vi "Operate.vi"(8 "error in (no error)":errorcluster, 11 "Multiply in":refnum<class "Multiply.lvclass">) -> (0 "error out":errorcluster, 2 "C":dbl, 3 "Multiply out":refnum<class "Multiply.lvclass">)   [LabVIEW 2021, in "Calculator.lvlib" / "Multiply.lvclass"]
doc: "This VI is a method for multiply class."
uses:
  Multiply.lvclass
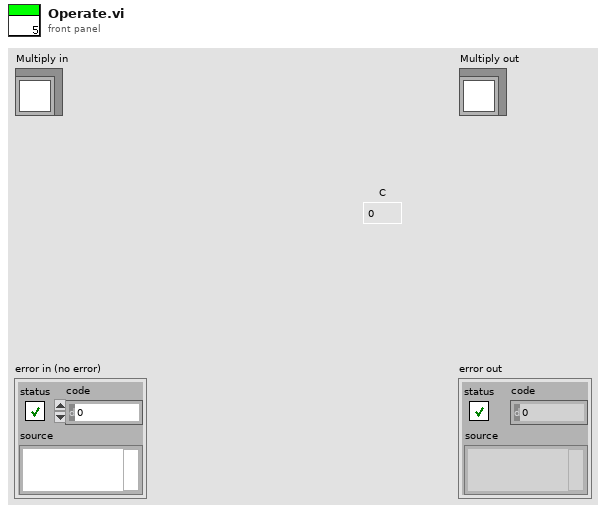
[diagram p1: front panel]
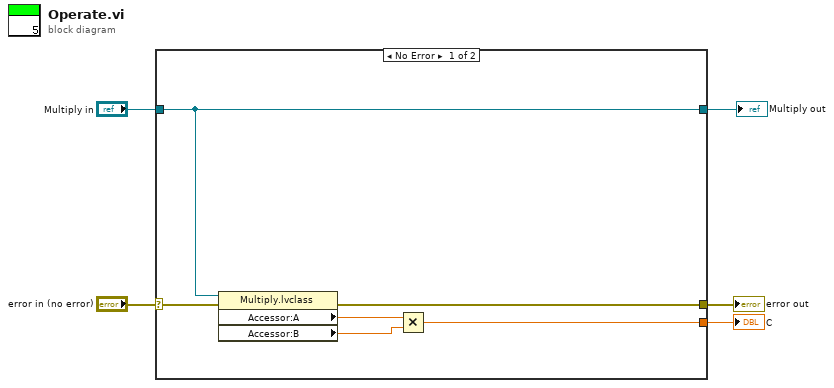
[diagram p0: block diagram]
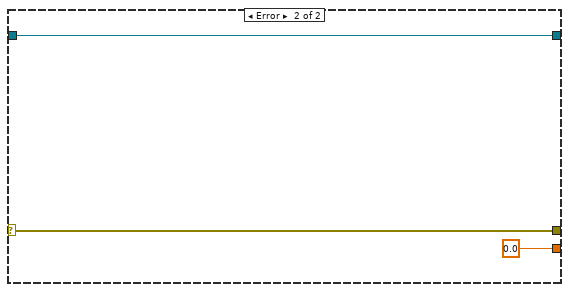
[diagram p2: hidden frame]
diagram:
  n1 = case shown="No Error" "error in (no error)" {
    selector: "error in (no error)" -> [w10 w14]
    tunnel: [w9 w14] -> w4
    tunnel: [w8 w13] -> w2
    tunnel: "Multiply in" -> [w8 w13]
    tunnel: [w11 0.0] -> w1
    frame No Error {
      n2 = property class="Multiply.lvclass"(reference=w8, error in=w10) -> (error out=w9:errorcluster, "Accessor:A"=w7:dbl, "Accessor:B"=w6:dbl)  [unwired: 1 out]
      n3 = Multiply(x=w7, y=w6) -> (x*y=w11:dbl)
    }
    frame Error {
    }
  }
  "error out" <- w4
  "Multiply out" <- w2
  "C" <- w1
